vi "validate configuration.vi"(8 "error in":errorcluster, 11 "EthernetIP configuration in":refnum<class "EthernetIP configuration.lvclass">) -> (0 "error out":errorcluster, 3 "EthernetIP configuration out":refnum<class "EthernetIP configuration.lvclass">)   [LabVIEW 2013, in "EthernetIP configuration.lvclass"]
doc: "This function performs validation of the configuration. This function should be safe to call at any point and should not rely on anything in the runtime environment."
uses:
  EthernetIP configuration.lvclass
  <vilib>/NI/Tag Bus Module Framework/module configuration/TBM module configuration.lvclass
  EthernetIP configuration.lvclass/EthernetIP configuration.ctl
  channel/EthernetIP Channel.lvclass/EthernetIP Channel.ctl
  <vilib>/NI/Tag Bus/tag/tag descriptor.lvclass/tag descriptor.ctl
  channel/Read Instance ID.vi
  channel/Read byte index.vi
  <vilib>/NI/Tag Bus/tag/read data type.vi
  <vilib>/NI/Tag Bus/tag/read tag name.vi
  <vilib>/NI/Tag Bus Module Framework/root configuration/TBM configuration.lvclass
  channel/EthernetIP Channel.lvclass
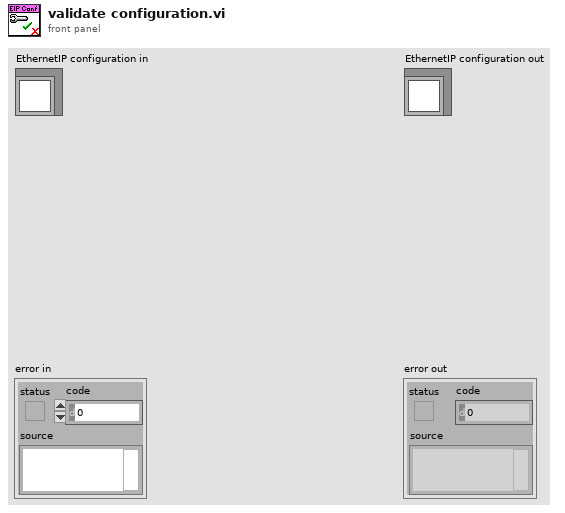
[diagram p1: front panel]
types:
  T1 = typedef "EthernetIP configuration.lvclass/assembly definition.ctl" = cluster{"name":string, "Instance ID":u32, "Type":T2, "Size (elements)":u32, "big endian?":bool, "data type":T3}
  T2 = typedef "EthernetIP configuration.lvclass/assembly type.ctl" = enum32{"Producing", "Consuming"}
  T3 = typedef "tag bus.lvlib/tag descriptor.lvclass/Data Type.ctl" = enum16{"Double", "Single", "I64", "I32", "I16", "I8", "U64", "U32", "U16", "U8", "Boolean", "String", "Array of Double", "Array of Single", "Array of I64", "Array of I32", "Array of I16", "Array of I8", "Array of U64", "Array of U32", "Array of U16", "Array of U8", "Array of Boolean", "Array of String"}
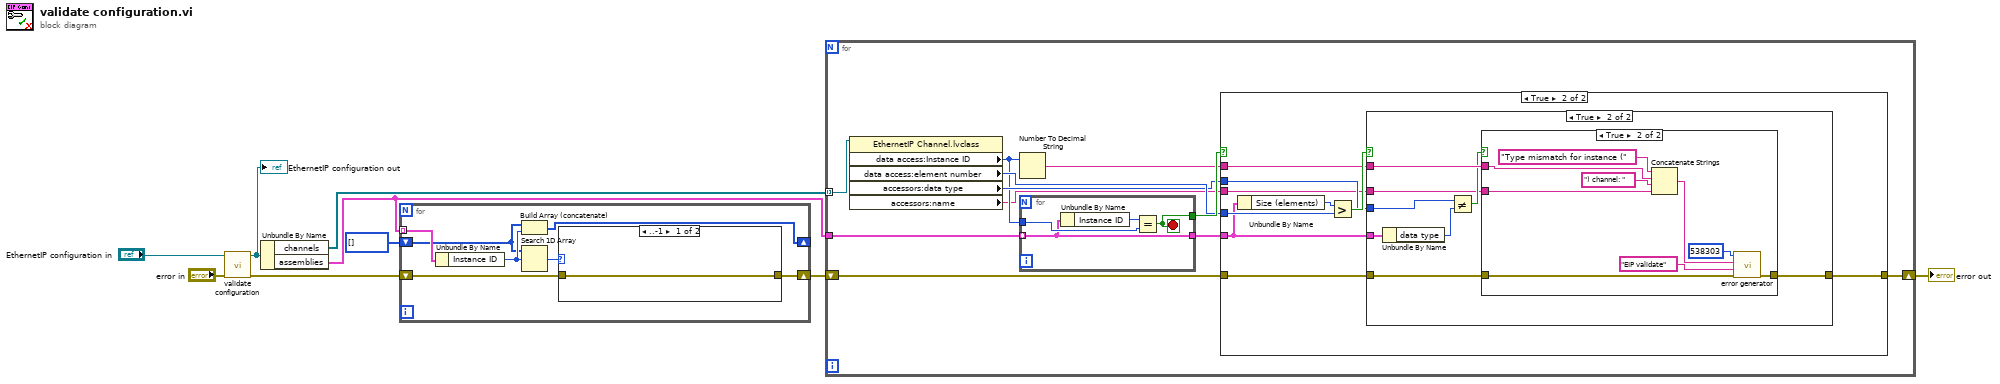
[diagram p0: block diagram]
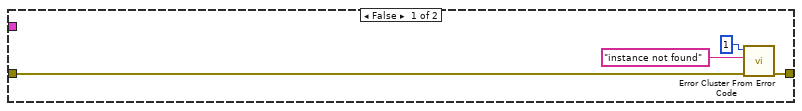
[diagram p2: hidden frame]
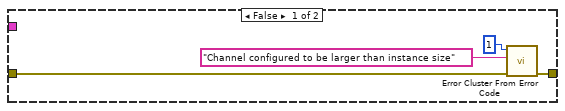
[diagram p3: hidden frame]
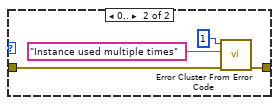
[diagram p5: hidden frame]
diagram:
  n1 = call-parent "validate configuration.vi"("error in"="error in", "configuration in"="EthernetIP configuration in") -> ("error out"=w5:errorcluster, "configuration out"=w7:refnum<class "EthernetIP configuration.lvclass">)  [unwired: 8 in]
  "EthernetIP configuration out" <- w7
  n2 = Unbundle By Name(w7) -> ("channels"=w4:refnum<class "EthernetIP Channel.lvclass">[], "assemblies"=w3:T1[])
  n3 = for {
    tunnel: w3 -> [w16] mode=indexing
    shift-right: [w15] -> _
    shift-left: u32[] [] -> [w13]
    shift-right: [w11] -> w2
    shift-left: w5 -> [w12]
    n4 = Unbundle By Name(w16) -> ("Instance ID"=w14:u32)
    n5 = Build Array (concatenate)(w13, w14) -> (w15:u32[])
    n6 = Search 1D Array(1D array=w13, element=w14) -> (index of element=w10:i32)  [unwired: 1 in]
    n7 = case shown="..-1" w10 {
      tunnel: w12 -> [w17 w20]
      tunnel: [w17 w21] -> w11
      frame ..-1 {
      }
      frame 0.. {
        n8 = call <vilib>:"Error Cluster From Error Code.vi"("error in (no error)"=w20, "error message (\"\")"="Instance used multiple times" ("error message (\"\")"), "error code (0)"=1) -> ("error out"=w21:errorcluster)  [unwired: 6 in]
      }
    }
  }
  n9 = for {
    tunnel: w4 -> [w31] mode=indexing
    tunnel: w3 -> [w32]
    shift-right: [w27] -> w1
    shift-left: w2 -> [w28]
    n10 = property class="EthernetIP Channel.lvclass"(reference=w31) -> ("data access:Instance ID"=w24:u32, "data access:element number"=w26:i32, "accessors:data type"=w25:T3, "accessors:name"=w22:string)  [unwired: 1 in, 2 out]
    n11 = Number To Decimal String(number=w24) -> (decimal integer string=w23:string)  [unwired: 1 in]
    n12 = for {
      tunnel: w32 -> [w69] mode=indexing
      tunnel: w24 -> [w70]
      tunnel: [w69] -> w29
      tunnel: [w68] -> w30
      stop <- w68 stop-if-true
      n13 = Unbundle By Name(w69) -> ("Instance ID"=w71:u32)
      n14 = Equal?(x=w71, y=w70) -> (x = y?=w68:bool)
    }
    n15 = case shown="True" w30 {
      tunnel: w29 -> [_ w40]
      tunnel: w28 -> [w35 w41]
      tunnel: [w34 w42] -> w27
      tunnel: w26 -> [_ w44]
      tunnel: w25 -> [_ w39]
      tunnel: w23 -> [_ w38]
      tunnel: w22 -> [_ w37]
      frame False {
        n16 = call <vilib>:"Error Cluster From Error Code.vi"("error in (no error)"=w35, "error message (\"\")"="instance not found" ("error message (\"\")"), "error code (0)"=1) -> ("error out"=w34:errorcluster)  [unwired: 6 in]
      }
      frame True {
        n17 = Unbundle By Name(w40) -> ("Size (elements)"=w45:u32)
        n18 = Greater?(x=w45, y=w44) -> (0:w43:bool)
        n19 = case shown="True" w43 {
          tunnel: [w46 w54] -> w42
          tunnel: w41 -> [w47 w53]
          tunnel: w40 -> [_ w57]
          tunnel: w39 -> [_ w55]
          tunnel: w38 -> [_ w52]
          tunnel: w37 -> [_ w50]
          frame False {
            n20 = call <vilib>:"Error Cluster From Error Code.vi"("error in (no error)"=w47, "error message (\"\")"="Channel configured to be larger than instance size" ("error message (\"\")"), "error code (0)"=1) -> ("error out"=w46:errorcluster)  [unwired: 6 in]
          }
          frame True {
            n21 = Unbundle By Name(w57) -> ("data type"=w56:T3)
            n22 = Not Equal?(x=w55, y=w56) -> (x != y?=w51:bool)
            n23 = case shown="True" w51 {
              tunnel: [w58 w67] -> w54
              tunnel: w53 -> [w58 w66]
              tunnel: w52 -> [_ w63]
              tunnel: w50 -> [_ w59]
              frame False {
              }
              frame True {
                n24 = Concatenate Strings("Type mismatch for instance (" ("string"), w63, ") channel: " ("string"), w59) -> (w62:string)
                n25 = call <vilib>:"error generator.vi"("error in"=w66, "source"="EIP validate", "append error message"=w62, "error code (0)"=538303) -> ("error out"=w67:errorcluster)  [unwired: 7 in]
              }
            }
          }
        }
      }
    }
  }
  "error out" <- w1
